vi "Kinesis - KBD101 - Get Status Bits.vi"() -> ()   [LabVIEW 2019]
doc: "Shows how to set and get stage axis info parameters for a motor channel."
uses:
  C:/Program Files (x86)/National Instruments/LabVIEW 2019/user.lib/ThorKDC101/Kinesis_with_LabVIEW_Examples_LV12 - v3/Thorlabs.MotionControl.Controls.dll
  Thorlabs.MotionControl.Controls.dll
  C:/Program Files (x86)/National Instruments/LabVIEW 2019/user.lib/ThorKDC101/Kinesis_with_LabVIEW_Examples_LV12 - v3/Thorlabs.MotionControl.KCube.BrushlessMotorCLI.dll
  Thorlabs.MotionControl.KCube.BrushlessMotorCLI.dll
panel:
  in  "stop":bool
  out "1":bool
  out "2":bool
  out "3":bool
  out "4":bool
  out "5":bool
  out "6":bool
  out "7":bool
  out "8":bool
  out "9":bool
  out "10":bool
  out "11":bool
  out "12":bool
  out "13":bool
  out "14":bool
  out "15":bool
  out "16":bool
  out "17":bool
  out "18":bool
  out "19":bool
  out "20":bool
  out "21":bool
  out "22":bool
  out "23":bool
  out "24":bool
  out "25":bool
  out "26":bool
  out "27":bool
  out "28":bool
  out "29":bool
  out "30":bool
  out "31":bool
  out "32":bool
  in  "Serial Number":string
  in  "KCubeBrushlessControl":refnum<k24>(container)
  # "Notes:"
  # "- Ensure that the appropriate .DLLs are copied into your Project Folder. Check that the correct bit type are used depending on your version of LabVIEW\ni.e. 32-bit or 64-bit.\n\n\n\n\n\n\n\n\n\n\n\n\n\n\n- Open the example VI through the LabVIEW Project Explorer to correctly load the User Interface from Thorlabs.MotionControl.Controls.dll."
  # "Thorlabs Hardware: KBD101 - K-Cube Brushless DC Servo Motor Controller\n https://www.thorlabs.com/thorproduct.cfm?partnumber=KBD101\n\nDescription: This VI will enable you to communicate with KBD101 to control DC Brushless Stages. The VI will poll status bits, through use of the GetStatusBits method, every 250ms.\n\nInstructions: \n1) Connect your KBD101 device to your PC & power the device, ensuring your stage/actutator is connected. For full device setup, the device product manual can be found on our website here. - https://www.thorlabs.com/thorproduct.cfm?partnumber=KBD101\n2) Enter the device serial number below.\n3) Click 'Run' in the LabVIEW Toolbar.\n4) To end the Program click 'END PROGRAM'"
  # "Example Image of .NET Controller - VI opened via Project Explorer/ not opened via Project Explorer"
  # "VI Not Opened via Project Explorer"
  # "VI Opened via Project Explorer"
  # "- To explore the range of methods available, please visit the .NET API, included with your Kinesis software.\n\n- For tips on building your own VIs with Thorlabs Motion Control Hardware, please see our LabVIEW Guide here.\nhttps://www.thorlabs.com/newgrouppage9.cfm?objectgroup_id=10285"
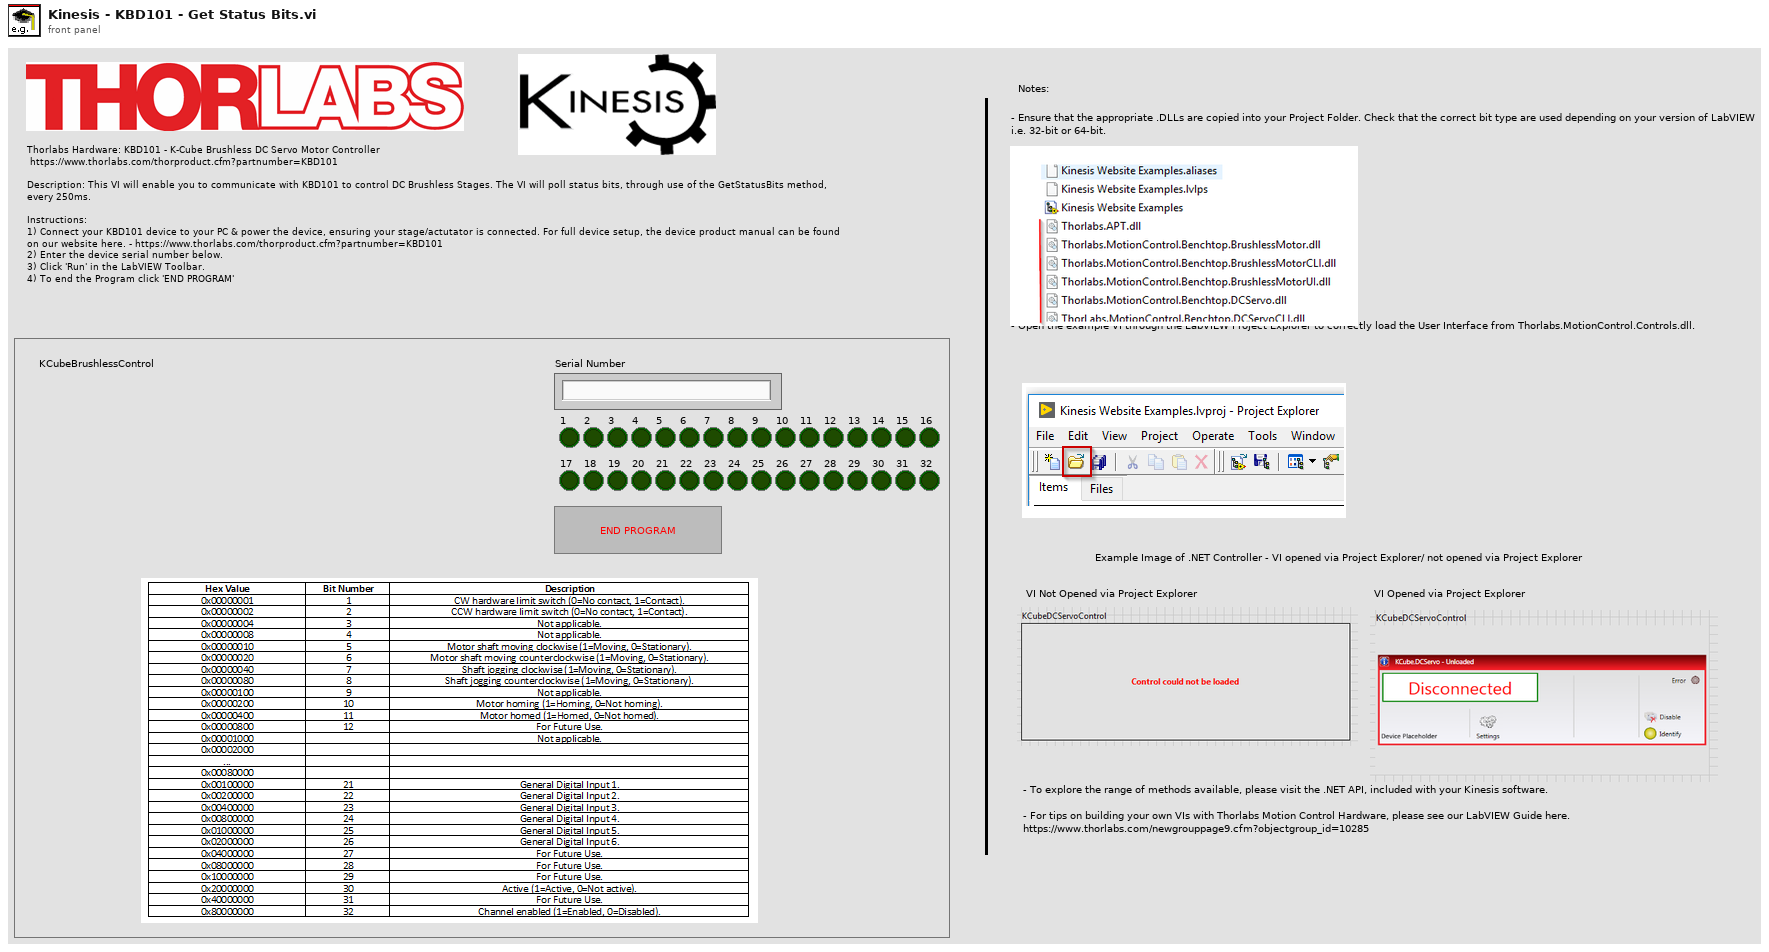
[diagram p1: front panel]
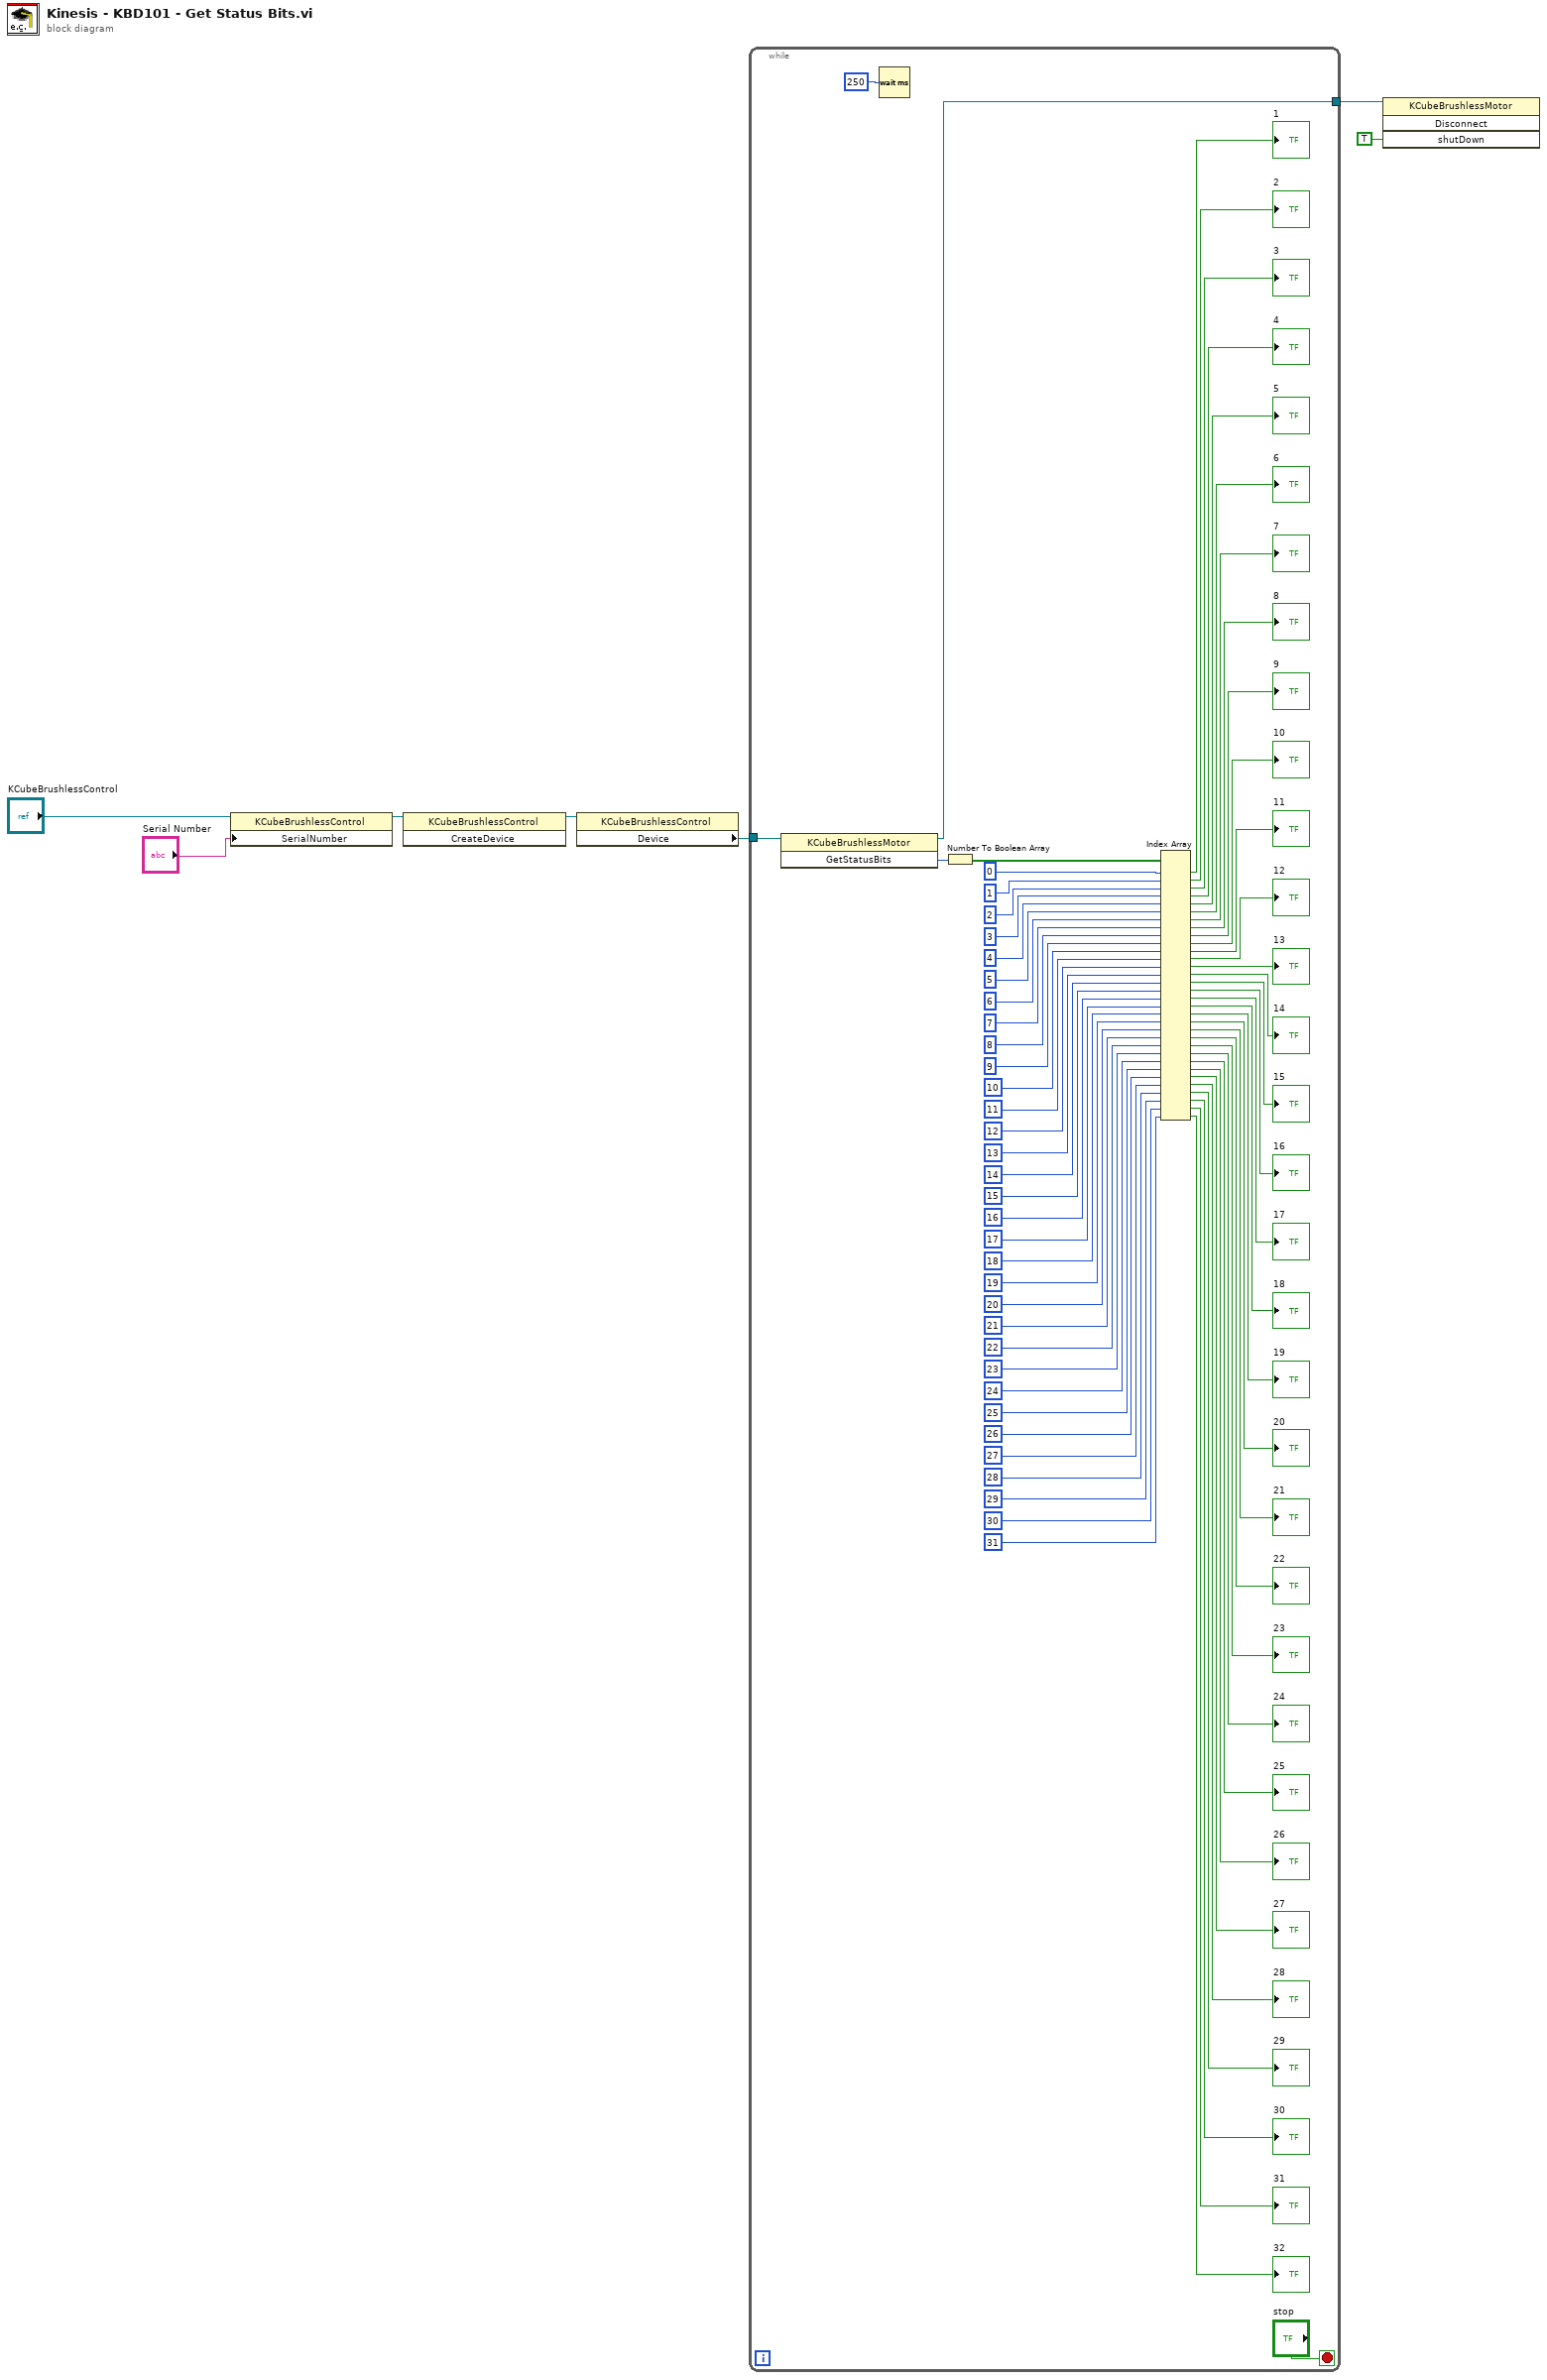
[diagram p0: block diagram]
diagram:
  n1 = property class="KCubeBrushlessControl"(reference="KCubeBrushlessControl", "SerialNumber"="Serial Number") -> (reference out=w6:refnum<k24>)  [unwired: 1 in, 1 out]
  n2 = invoke class="KCubeBrushlessControl" method="CreateDevice"(reference=w6) -> (reference out=w5:refnum<k24>)  [unwired: 2 in, 2 out]
  n3 = property class="KCubeBrushlessControl"(reference=w5) -> ("Device"=w2:refnum<k24>)  [unwired: 1 in, 2 out]
  n4 = while {
    tunnel: w2 -> [w77]
    tunnel: [w8] -> w1
    stop <- "stop" stop-if-true
    n5 = invoke class="KCubeBrushlessMotor" method="GetStatusBits"(reference=w77) -> (reference out=w8:refnum<k24>, "GetStatusBits"=w10:u32)  [unwired: 2 in, 1 out]
    n6 = Wait (ms)(milliseconds to wait=u32 250) -> ()  [unwired: 1 out]
    n7 = Number To Boolean Array(number=w10) -> (Boolean array=w11:bool[])
    n8 = Index Array(array=w11, index #1=0 ("index"), index #2=1 ("index"), index #3=2 ("index"), index #4=3 ("index"), index #5=4 ("index"), index #6=5 ("index"), index #7=6 ("index"), index #8=7 ("index"), index #9=8 ("index"), index #10=9 ("index"), index #11=10 ("index"), index #12=11 ("index"), index #13=12 ("index"), index #14=13 ("index"), index #15=14 ("index"), index #16=15 ("index"), index #17=16 ("index"), index #18=17 ("index"), index #19=18 ("index"), index #20=19 ("index"), index #21=20 ("index"), index #22=21 ("index"), index #23=22 ("index"), index #24=23 ("index"), index #25=24 ("index"), index #26=25 ("index"), index #27=26 ("index"), index #28=27 ("index"), index #29=28 ("index"), index #30=29 ("index"), index #31=30 ("index"), index #32=31 ("index")) -> (element #1=→"1":bool, element #2=→"2":bool, element #3=→"3":bool, element #4=→"4":bool, element #5=→"5":bool, element #6=→"6":bool, element #7=→"7":bool, element #8=→"8":bool, element #9=→"9":bool, element #10=→"10":bool, element #11=→"11":bool, element #12=→"12":bool, element #13=→"13":bool, element #14=→"14":bool, element #15=→"15":bool, element #16=→"16":bool, element #17=→"17":bool, element #18=→"18":bool, element #19=→"19":bool, element #20=→"20":bool, element #21=→"21":bool, element #22=→"22":bool, element #23=→"23":bool, element #24=→"24":bool, element #25=→"25":bool, element #26=→"26":bool, element #27=→"27":bool, element #28=→"28":bool, element #29=→"29":bool, element #30=→"30":bool, element #31=→"31":bool, element #32=→"32":bool)
  }
  n9 = invoke class="KCubeBrushlessMotor" method="Disconnect"(reference=w1, "shutDown"=TRUE) -> ()  [unwired: 2 in, 4 out]
